vi "Get Decimation.vi"(11 "Timing in":refnum<class "Engine Timing.lvclass">) -> (2 "Decimation":u64=1, 3 "Timing out":refnum<class "Engine Timing.lvclass">)   [LabVIEW 2017, in "Data Sharing Framework Core.lvlib" / "Data Sharing Framework Engine.lvlib" / "Engine Timing.lvclass"]
uses:
  Engine Timing.lvclass
  Engine Timing.lvclass/Engine Timing.ctl
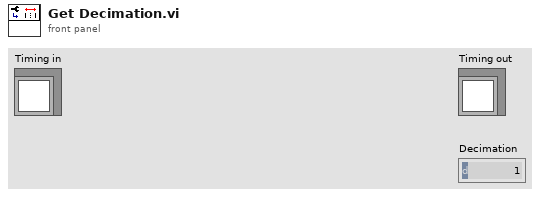
[diagram p1: front panel]
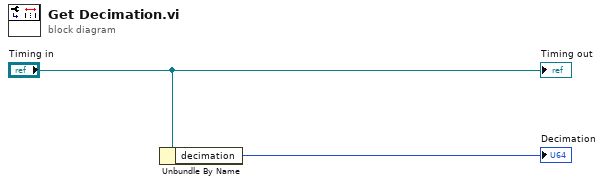
[diagram p0: block diagram]
diagram:
  n1 = Unbundle By Name("Timing in") -> ("decimation"=→"Decimation":u64)
  "Timing out" <- "Timing in"
